vi "Text_Create.vi"(7 "Object Attributes":T2, 8 "error in (no error)":errorcluster, 10 "Text Attributes":T1, 11 "Text In":refnum<class "Text.lvclass">) -> (0 "error out":errorcluster, 3 "Text Out":refnum<class "Text.lvclass">)   [LabVIEW 2015, in "Front Panel Publisher.lvlib" / "Text.lvclass"]
uses:
  Text.lvclass
  Object_class/Attributes.ctl
  Object_class/Coordinates.ctl
  Attributes.ctl
  Object_class/Object.lvclass
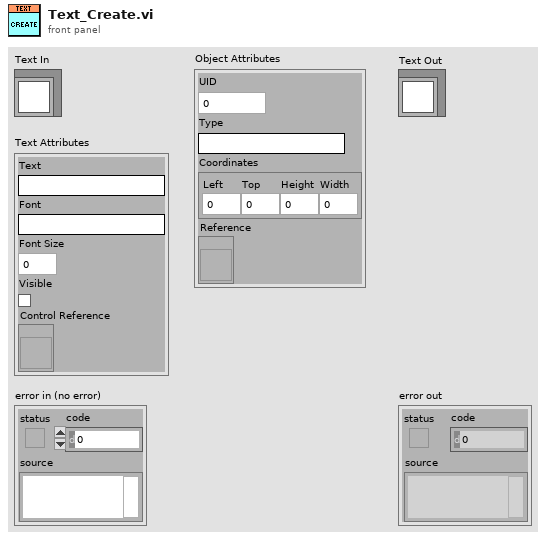
[diagram p1: front panel]
types:
  T1 = typedef "Front Panel Publisher.lvlib/Text.lvclass/Attributes.ctl" = cluster{"Text":string, "Font":string, "Font Size":u32, "Visible":bool, "Control Reference":refnum<vi>}
  T2 = typedef "Front Panel Publisher.lvlib/Object.lvclass/Attributes.ctl" = cluster{"UID":i32, "Type":string, "Coordinates":T3, "Reference":refnum<vi>}
  T3 = typedef "Front Panel Publisher.lvlib/Object.lvclass/Coordinates.ctl" = cluster{"Left":i32, "Top":i32, "Height":u32, "Width":u32}
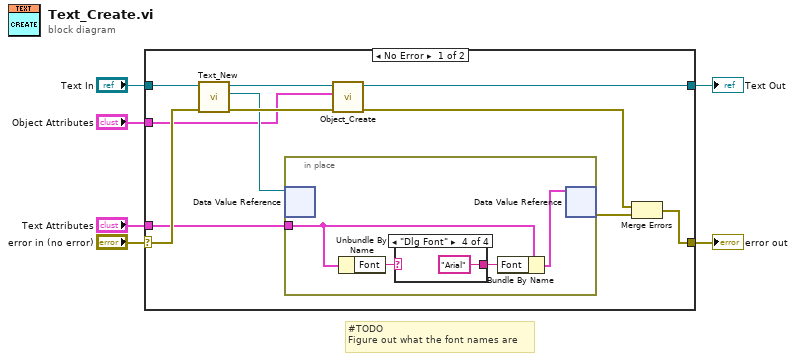
[diagram p0: block diagram]
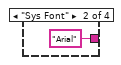
[diagram p3: hidden frame]
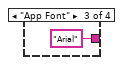
[diagram p4: hidden frame]
diagram:
  # "#TODO\nFigure out what the font names are"
  n1 = case shown="No Error" "error in (no error)" {
    selector: "error in (no error)" -> [w16 w27]
    tunnel: [w14 w27] -> w5
    tunnel: "Text In" -> [w17 w26]
    tunnel: [w11 w26] -> w3
    tunnel: "Object Attributes" -> [w7 _]
    tunnel: "Text Attributes" -> [w8 _]
    frame No Error {
      n2 = call "Text_New.vi"("error in (no error)"=w16, "Text In"=w17) -> ("error out"=w12:errorcluster, "DVRRefOut"=w10:refnum<data-value>, "Text Out"=w13:refnum<class "Text.lvclass">)  [unwired: 6 in, 1 out]
      n3 = in-place {
        in-place-border: w8 -> [w20]
        n4 = in-place-dvr #1(w10) -> ()  [unwired: 2 out]
        n5 = Unbundle By Name(w20) -> ("Font"=w21:string)
        n6 = case shown="\"Dlg Font\"" w21 {
          selector: w21 -> [w22 _ _ _]
          tunnel: [w22 "Arial" "Arial" "Arial"] -> w18
          frame Default {
          }
          frame "Sys Font" {
          }
          frame "App Font" {
          }
          frame "Dlg Font" {
          }
        }
        n7 = Bundle By Name(cluster=w20, "Font"=w18) -> (w19:T1)
        n8 = in-place-dvr #1(w19) -> (w15:errorcluster)  [unwired: 1 out]
      }
      n9 = call "Object_Create.vi"("error in (no error)"=w12, "Object Attributes"=w7, "Object In"=w13) -> ("error out"=w9:errorcluster, "Object Out"=w11:refnum<class "Text.lvclass">)  [unwired: 7 in]
      n10 = Merge Errors(w9, w15) -> (w14:errorcluster)
    }
    frame Error {
    }
  }
  "error out" <- w5
  "Text Out" <- w3
